vi "ELVIS III v1.0 Reserve DO Block.vi"(7 "Allow multiple opens?":bool, 8 "error in (no error)":errorcluster, 10 "DO (N Samples) Channel List":T2, 11 "Generic FPGA Reference":T1) -> (0 "error out":errorcluster)   [LabVIEW 2021]
uses:
  <vilib>/myRIO/Common/Instrument Driver Framework/myRIO v1.0/DO Block/typedefs/DO Block Channels List.ctl
  <vilib>/myRIO/Common/Instrument Driver Framework/myRIO v1.0/DO Block/typedefs/DO Block Channels Enum.ctl
  <vilib>/myRIO/Common/Instrument Driver Framework/Utilities/typedefs/Generic FPGA Reference.ctl
  <vilib>/myRIO/Common/Instrument Driver Framework/ELVIS III v1.0/Resource Manager/vis/ELVIS III v1.0 Create Configuration List.vi
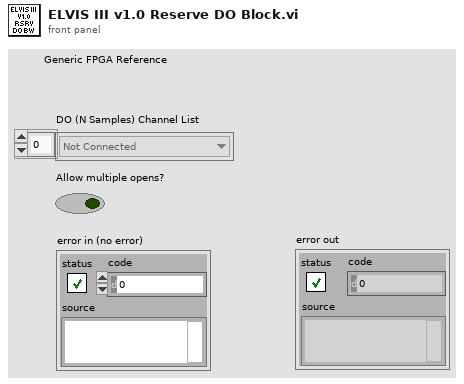
[diagram p1: front panel]
types:
  T1 = typedef "Generic FPGA Reference.ctl" = refnum<k20>
  T2 = typedef "DO Block Channels List.ctl" = T3[]
  T3 = typedef "DO Block Channels Enum.ctl" = enum16{"Not Connected", "A/DO0 (N Samples)", "A/DO1 (N Samples)", "A/DO2 (N Samples)", "A/DO3 (N Samples)", "A/DO4 (N Samples)", "A/DO5 (N Samples)", "A/DO6 (N Samples)", "A/DO7 (N Samples)", "A/DO8 (N Samples)", "A/DO9 (N Samples)", "A/DO10 (N Samples)", "A/DO11 (N Samples)", "A/DO12 (N Samples)", "A/DO13 (N Samples)", "A/DO14 (N Samples)", "A/DO15 (N Samples)", "A/DO16 (N Samples)", "A/DO17 (N Samples)", "A/DO18 (N Samples)", "A/DO19 (N Samples)", "B/DO0 (N Samples)", "B/DO1 (N Samples)", "B/DO2 (N Samples)", "B/DO3 (N Samples)", "B/DO4 (N Samples)", "B/DO5 (N Samples)", "B/DO6 (N Samples)", "B/DO7 (N Samples)", "B/DO8 (N Samples)", "B/DO9 (N Samples)", "B/DO10 (N Samples)", "B/DO11 (N Samples)", "B/DO12 (N Samples)", "B/DO13 (N Samples)", "B/DO14 (N Samples)", "B/DO15 (N Samples)", "B/DO16 (N Samples)", "B/DO17 (N Samples)", "B/DO18 (N Samples)", "B/DO19 (N Samples)"}
  T4 = typedef "ELVIS III v1.0 Channel Reservation List.ctl" = T5[]
  T5 = typedef "ELVIS III v1.0 Channel Reservation Info.ctl" = cluster{"Channel Name":string, "Connector":T6, "MutexIDs":u32[]}
  T6 = typedef "ELVIS III v1.0 Connector List.ctl" = enum32{"None", "ConnectorA", "ConnectorB"}
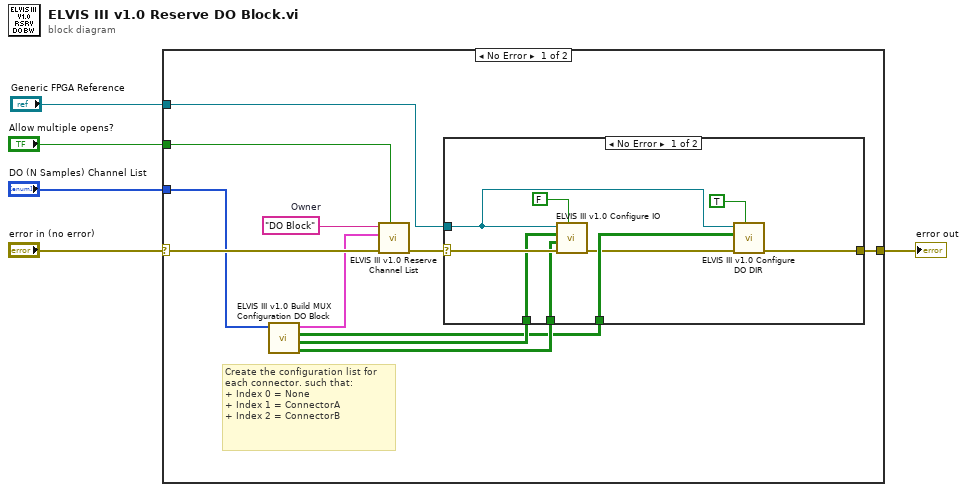
[diagram p0: block diagram]
diagram:
  n1 = case shown="No Error" "error in (no error)" {
    selector: "error in (no error)" -> [w15 w27]
    tunnel: "DO (N Samples) Channel List" -> [w12 _]
    tunnel: [w10 w27] -> w4
    tunnel: "Allow multiple opens?" -> [w16 _]
    tunnel: "Generic FPGA Reference" -> [w6 _]
    frame No Error {
      w14 = "DO Block"  # Owner
      # "Create the configuration list for each connector. such that:\n+ Index 0 = None\n+ Index 1 = ConnectorA\n+ Index 2 = ConnectorB"
      n2 = call <vilib>:"ELVIS III v1.0 Build MUX Configuration DO Block.vi"("DO (N Samples) Channel List"=w12) -> ("Configuration Bitmask Array"=w8:bool[][], "Configration Bitcode Array"=w9:bool[][], "DIO Mode Bitmask"=w7:bool[][], "Channel Reservation List"=w13:T4)  [unwired: 7 in]
      n3 = call <vilib>:"ELVIS III v1.0 Reserve Channel List.vi"("Allow multiple opens?"=w16, "error in (no error)"=w15, "Channel Reservation List"=w13, "Owner"=w14) -> ("error out"=w11:errorcluster)  [unwired: 7 in]
      n4 = case shown="No Error" w11 {
        selector: w11 -> [w25 w26]
        tunnel: w6 -> [w17 _]
        tunnel: [w18 w26] -> w10
        tunnel: w9 -> [w24 _]
        tunnel: w8 -> [w23 _]
        tunnel: w7 -> [w21 _]
        frame No Error {
          n5 = call <vilib>:"ELVIS III v1.0 Configure IO.vi"("Value"=FALSE, "error in (no error)"=w25, "Bitmask Array"=w23, "Bitcode Array"=w24, "myRIO FPGA Ref In"=w17) -> ("error out"=w19:errorcluster)  [unwired: 6 in]
          n6 = call <vilib>:"ELVIS III v1.0 Configure DO DIR.vi"("Apply Bitmask?"=TRUE, "error in (no error)"=w19, "Bitmask Array"=w21, "myRIO FPGA Ref In"=w17) -> ("error out"=w18:errorcluster)  [unwired: 7 in]
        }
        frame Error {
        }
      }
    }
    frame Error {
    }
  }
  "error out" <- w4
